vi "validate gen against lvgen.vi"() -> ()   [LabVIEW 2014]
uses:
  generate string.vi
  escape json string.vi
  json generator.lvlib
panel:
  out "escaped":string
  out "broke":bool
  out "original":string
  out "escape":dbl
  out "unescp":dbl
  out "unescaped":string
  # "Theirs*:\n0.0341413\n0.0389397\n*nulls cause failure (ie \\00, not \"null\")"
  # "Mine:\n0.0145317\n0.0205341"
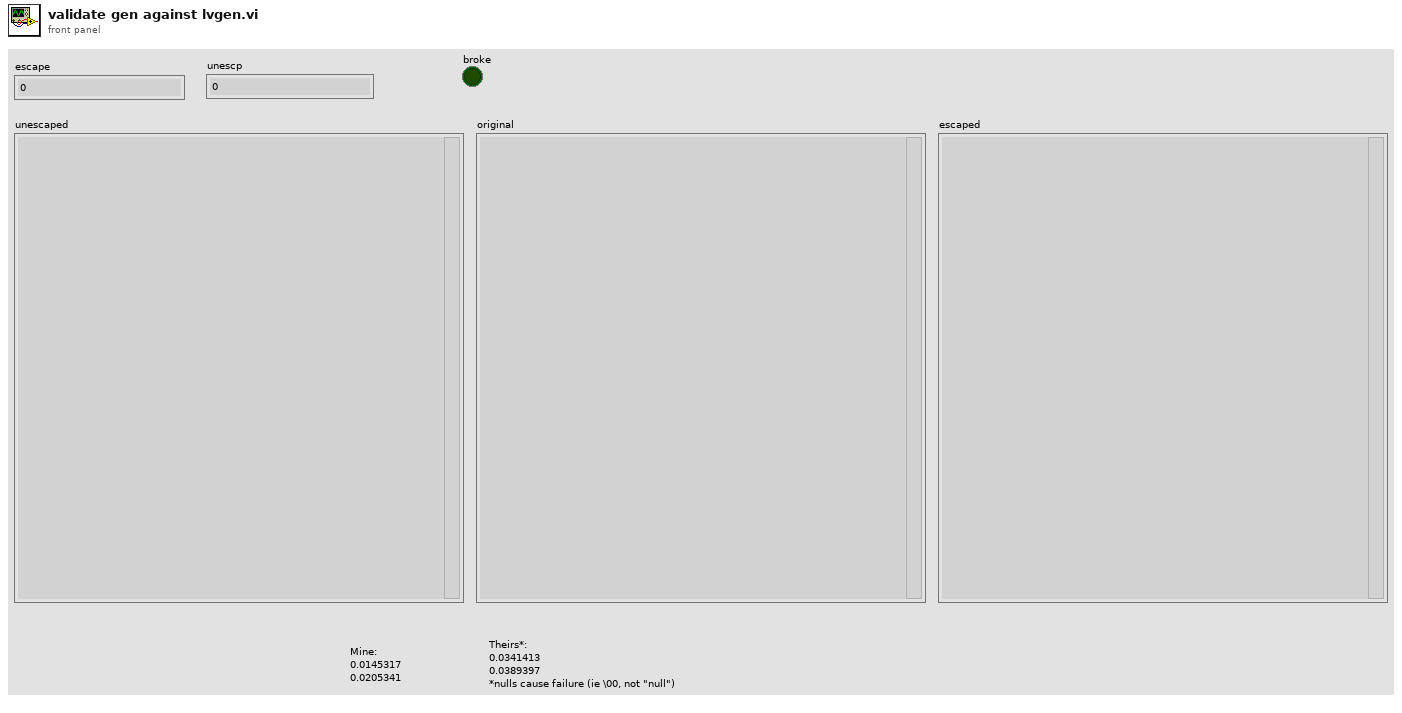
[diagram p1: front panel]
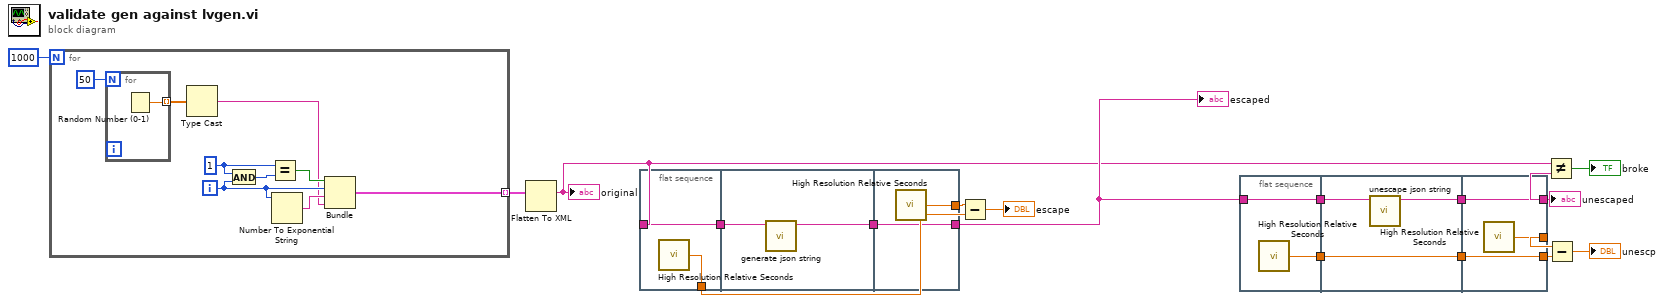
[diagram p0: block diagram]
diagram:
  n1 = for {
    N: 1000 -> [_]
    tunnel: [w22] -> w17 mode=indexing
    i -> [w26]
    w24 = 1 ("x")
    n2 = for {
      N: 50 -> [_]
      tunnel: [w28] -> w21 mode=indexing
      n3 = Random Number (0-1)() -> (number: 0 to 1=w28:dbl)
    }
    n4 = Type Cast(x=w21) -> (*(type *) &x=w19:string)  [unwired: 1 in]
    n5 = And(x=w24, y=w26) -> (x .and. y?=w25:i32)
    n6 = Equal?(x=w24, y=w25) -> (x = y?=w23:bool)
    n7 = Number To Exponential String(number=w26) -> (E-format string=w27:string)  [unwired: 3 in]
    n8 = Bundle(w23, w26, w27, w19) -> (w22:cluster{bool, i32, string, string})  [unwired: 1 in]
  }
  n9 = Flatten To XML(anything=w17) -> (xml string=w2:string)
  "original" <- w2
  n10 = flat-sequence {
    tunnel: w2 -> [w30]
    tunnel: [w30] -> w7
    tunnel: [w29] -> w5
    tunnel: [w32] -> w8
    tunnel: w7 -> [w31]
    tunnel: [w34] -> w9
    tunnel: w8 -> [w34]
    tunnel: [w33] -> w6
    frame #0 {
      n11 = call <vilib>:"High Resolution Relative Seconds.vi"() -> ("relative seconds"=w29:dbl)
    }
    frame #1 {
      n12 = call-poly "generate json string.vi"("base string"=w31) -> ("json string"=w32:string)  [unwired: 10 in]
    }
    frame #2 {
      n13 = call <vilib>:"High Resolution Relative Seconds.vi"() -> ("relative seconds"=w33:dbl)
    }
  }
  n14 = Subtract(x=w6, y=w5) -> (x-y=→"escape":dbl)
  n15 = flat-sequence {
    tunnel: [w36] -> w16
    tunnel: w9 -> [w36]
    tunnel: [w35] -> w13
    tunnel: w16 -> [w38]
    tunnel: [w37] -> w15
    tunnel: w13 -> [w39]
    tunnel: [w39] -> w12
    tunnel: [w42] -> w3
    tunnel: w15 -> [w42]
    tunnel: [w41] -> w14
    tunnel: w12 -> [w40]
    tunnel: [w40] -> w11
    frame #0 {
      n16 = call <vilib>:"High Resolution Relative Seconds.vi"() -> ("relative seconds"=w35:dbl)
    }
    frame #1 {
      n17 = call "unescape json string.vi"("base string"=w38) -> ("String out"=w37:string)  [unwired: 10 in]
    }
    frame #2 {
      n18 = call <vilib>:"High Resolution Relative Seconds.vi"() -> ("relative seconds"=w41:dbl)
    }
  }
  n19 = Not Equal?(x=w2, y=w3) -> (x != y?=→"broke":bool)
  n20 = Subtract(x=w14, y=w11) -> (x-y=→"unescp":dbl)
  "unescaped" <- w3
  "escaped" <- w9
